vi "Vision Processing.vi"(4 "yaw":dbl, 6 "Line Border":cluster{"Top":dbl, "Bottom":dbl}={"Top"=6.0, "Bottom"=1.0}, 7 "LED Color":T5={"Hue"={107.81818389892578, 139.81818389892578}, "Sat"={176.07142857142858, 255.0}, "Val"={40.53571428571429, 255.0}} {"Hue" scale=0.0..255.0 scale format="%#_3g"}, 8 "Score Cutoff %":dbl=70.0, 9 "Masked Image":T1, 10 "Boiler?":bool, 11 "New Image":T1) -> (1 "Original Image":T1(plugin-control), 2 "Results":T4 {"Score" format="%#_3g"; "Pixels"."Rectangle"."Numeric 5" format="%#_3g"; "Pixels"."Rectangle"."Numeric 3" format="%#_3g"; "Pixels"."Rectangle"."Numeric 2" format="%#_3g"; "Pixels"."Rectangle"."Numeric" format="%#_3g"; "Normalized"."Rectangle"."Numeric 5" format="%#_2g"; "Normalized"."Rectangle"."Numeric 3" format="%#_2g"; "Normalized"."Rectangle"."Numeric 2" format="%#_2g"; "Normalized"."Rectangle"."Numeric" format="%#_2g"; "Normalized"."Center"."?" format="%#_3g"; "Normalized"."Center"."?" format="%#_3g"; "Distance (ft)" format="%#_3g"}, 3 "Mask":T1(plugin-control))   [LabVIEW 2016]
uses:
  Vision Support Code/Camera Types.ctl
  <vilib>/Rock Robotics/WPI/Camera/WPI_CameraImageSize.ctl
  <vilib>/vision/Image Controls.llb/IMAQ Image.ctl
  <vilib>/Rock Robotics/Network Tables/NT Write Number.vi
  <vilib>/Rock Robotics/Network Tables/NT Write Boolean.vi
  <vilib>/vision/NI_Vision_Development_Module.lvlib
panel:
  out "Edge?":bool
  out "Time":u32
  in  "Image Size":T2=enum."320x240"
  in  "Color Mode":u16(ring)=3 items=["RGB", "HSL", "HSV", "HSI"]
  in  "Particles":dbl=5.0
  in  "Camera Type":T3=enum."MS HD3000 640x480"
  out "Qualified Particles":i32
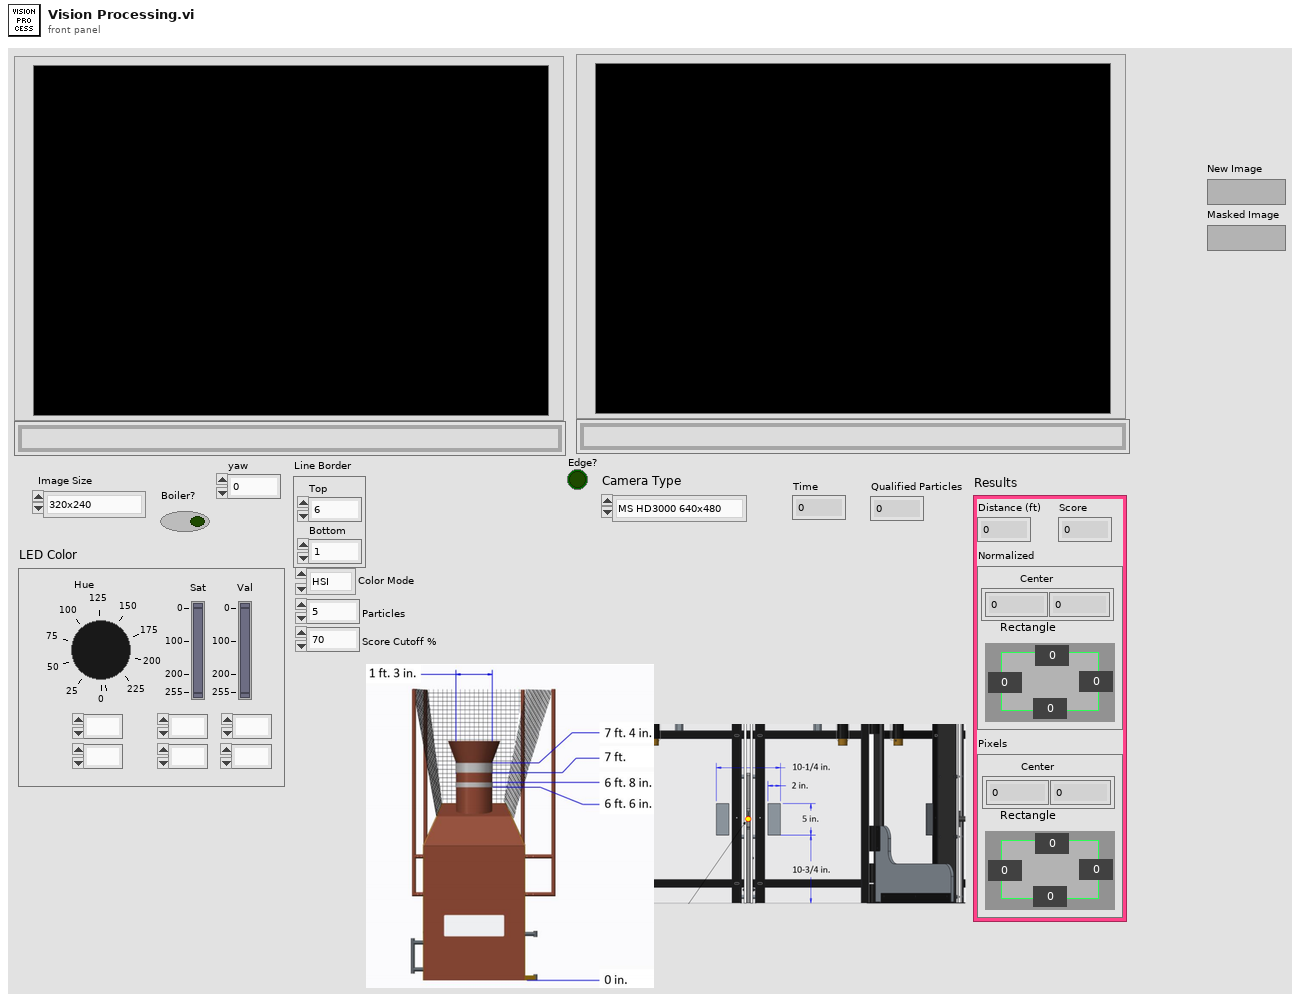
[diagram p1: front panel]
types:
  T1 = typedef "IMAQ Image.ctl" = refnum<image>
  T2 = typedef "WPI_CameraImageSize.ctl" = enum16{"640x480", "320x240", "160x120", "Custom"}
  T3 = typedef "Camera Types.ctl" = enum16{"206", "1011", "1013", "MS HD3000 square", "MS HD3000 640x480"}
  T4 = cluster{"Distance (ft)":dbl, "Score":dbl, "Normalized":cluster{"Center":cluster{dbl, dbl}, "Rectangle":cluster{"Numeric":dbl, "Numeric 2":dbl, "Numeric 3":dbl, "Numeric 5":dbl}}, "Pixels":cluster{"Center":cluster{dbl, dbl}, "Rectangle":cluster{"Numeric":dbl, "Numeric 2":dbl, "Numeric 3":dbl, "Numeric 5":dbl}}}
  T5 = cluster{"Hue":cluster{dbl, dbl}, "Sat":cluster{dbl, dbl}, "Val":cluster{dbl, dbl}}
  T6 = typedef "Particle Parameters" = i32
  T7 = cluster{"Left":dbl, "Top":dbl, "Right":dbl, "Bottom":dbl}
  T8 = cluster{"Distance (ft)":dbl, "Score":dbl, "Normalized":cluster{"Center":cluster{dbl, dbl}, "Rectangle":cluster{"Numeric":dbl, "Numeric 2":dbl, "Numeric 3":dbl, "Numeric 5":dbl}}, "Pixels":cluster{"Center":cluster{dbl, dbl}, "Rectangle":cluster{"Numeric":dbl, "Numeric 2":dbl, "Numeric 3":dbl, "Numeric 5":dbl}}}[]
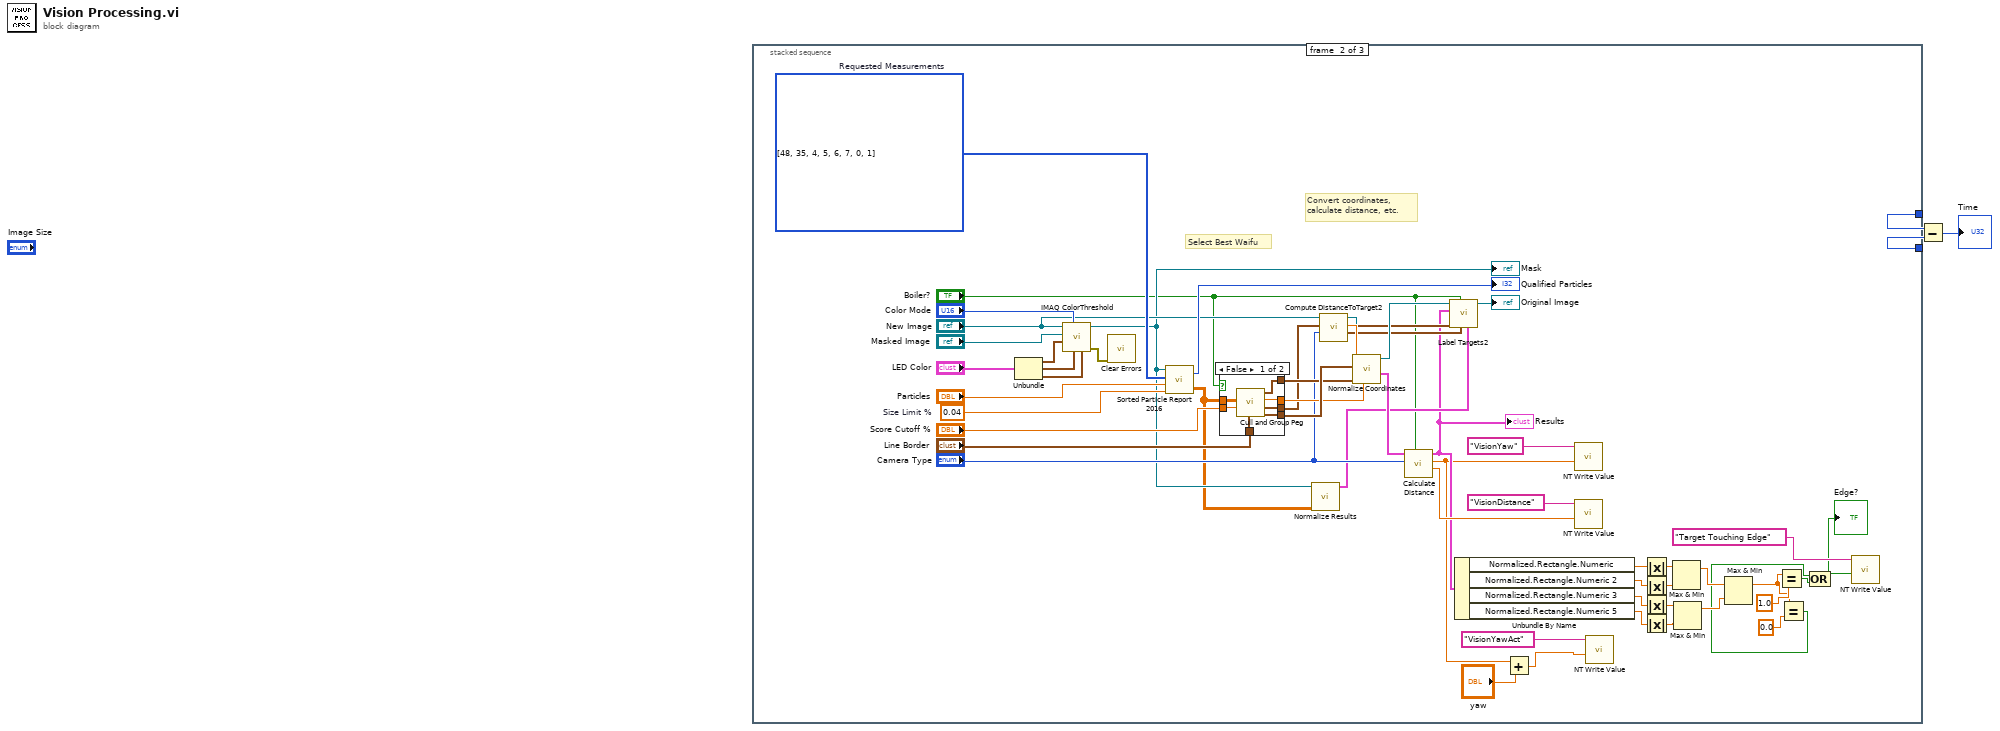
[diagram p0: block diagram]
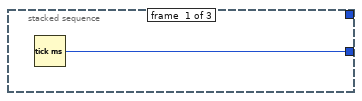
[diagram p2: hidden frame]
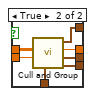
[diagram p3: hidden frame]
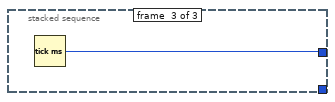
[diagram p4: hidden frame]
diagram:
  n1 = stacked-sequence {
    tunnel: [w4 _ _] -> w2
    tunnel: [_ _ w73] -> w3
    frame #0 {
      n2 = Tick Count (ms)() -> (millisecond timer value=w4:u32)
    }
    frame #1 {
      w39 = T6[] [48, 35, 4, 5, 6, 7, 0, 1] items=["Center of Mass X", "Center of Mass Y", "First Pixel X", "First Pixel Y", "Bounding Rect Left", "Bounding Rect Top", "Bounding Rect Right", "Bounding Rect Bottom", "Max Feret Diameter Start X", "Max Feret Diameter Start Y", "Max Feret Diameter End X", "Max Feret Diameter End Y", "Max Horiz. Segment Length Left", "Max Horiz. Segment Length Right", "Max Horiz. Segment Length Row", "-", "Bounding Rect Width", "Bounding Rect Height", "Bounding Rect Diagonal", "Perimeter", "Convex Hull Perimeter", "Holes' Perimeter", "Max Feret Diameter", "Equivalent Ellipse Major Axis", "Equivalent Ellipse Minor Axis", "Equivalent Ellipse Minor Axis (Feret)", "Equivalent Rect Long Side", "Equivalent Rect Short Side", "Equivalent Rect Diagonal", "Equivalent Rect Short Side (Feret)", "Average Horiz. Segment Length", "Average Vert. Segment Length", "Hydraulic Radius", "Waddel Disk Diameter", "-", "Area", "Holes' Area", "Particle & Holes' Area", "Convex Hull Area", "Image Area", "-", "Number of Holes", "Number of Horiz. Segments", "Number of Vert. Segments", "-", "Orientation", "Max Feret Diameter Orientation", "-", "% Area/Image Area", "% Area/(Particle & Holes' Area)", "Ratio of Equivalent Ellipse Axes", "Ratio of Equivalent Rect Sides", "-", "Elongation Factor", "Compactness Factor", "Heywood Circularity Factor", "Type Factor", "-", "Sum X", "Sum Y", "Sum XX", "Sum XY", "Sum YY", "Sum XXX", "Sum XXY", "Sum XYY", "Sum YYY", "-", "Moment of Inertia XX", "Moment of Inertia XY", "Moment of Inertia YY", "Moment of Inertia XXX", "Moment of Inertia XXY", "Moment of Inertia XYY", "Moment of Inertia YYY", "Norm. Moment of Inertia XX", "Norm. Moment of Inertia XY", "Norm. Moment of Inertia YY", "Norm. Moment of Inertia XXX", "Norm. Moment of Inertia XXY", "Norm. Moment of Inertia XYY", "Norm. Moment of Inertia YYY", "Hu Moment 1", "Hu Moment 2", "Hu Moment 3", "Hu Moment 4", "Hu Moment 5", "Hu Moment 6", "Hu Moment 7"]  # Requested Measurements
      w54 = 0.04  # Size Limit %
      # "Convert coordinates,\ncalculate distance, etc."
      # "Select Best Waifu"
      n3 = Unbundle("LED Color") -> ("Hue"=w58:cluster{dbl, dbl}, "Sat"=w57:cluster{dbl, dbl}, "Val"=w56:cluster{dbl, dbl})
      n4 = call "IMAQ ColorThreshold"("Blue or Luma or Val or Inten Range"=w56, "Green or Sat Range"=w57, "Color Mode"="Color Mode", "Red or Hue Range"=w58, "Image Dst"="Masked Image", "Image Src"="New Image") -> ("error out"=w53:errorcluster, "Image Dst Out"=w30:T1)  [unwired: 4 in]
      "Mask" <- w30
      n5 = call <vilib>:"Clear Errors.vi"("error in (no error)"=w53) -> ()  [unwired: 5 in, 2 out]
      n6 = call "Sorted Particle Report 2016.vi"("Min Area Size %"=w54, "Particle Count Limit"="Particles", "Pixel Measurements"=w39, "Image in"=w30) -> ("Sorted Data"=w29:dbl[][], "Particles"=→"Qualified Particles":i32)
      n7 = case shown="False" "Boiler?" {
        tunnel: "Score Cutoff %" -> [w64 w72]
        tunnel: [w59 w71] -> w50
        tunnel: [w62 w70] -> w46
        tunnel: [w61 w69] -> w45
        tunnel: [w60 w68] -> w42
        tunnel: "Line Border" -> [w65 w67]
        tunnel: w29 -> [w63 w66]
        frame False {
          n8 = call "Cull and Group Peg.vi"("Line Border"=w65, "Score Cutoff"=w64, "Sorted Data"=w63) -> ("Rect"=w59:T7, "Line"=w60:T7, "Score"=w61:dbl, "Center"=w62:cluster{"X":dbl, "Y":dbl})  [unwired: 5 in]
        }
        frame True {
          n9 = call "Cull and Group.vi"("Line Border"=w67, "Score Cutoff"=w72, "Sorted Data"=w66) -> ("Rect"=w71:T7, "Line"=w68:T7, "Score"=w69:dbl, "Center"=w70:cluster{"X":dbl, "Y":dbl})  [unwired: 5 in]
        }
      }
      n10 = call "Normalize Results.vi"("Sorted Data"=w29, "Image in"=w30) -> ("Results"=w28:T8)  [unwired: 9 in]
      n11 = call "Compute DistanceToTarget2.vi"("Camera Type"="Camera Type", "Line"=w42, "Image Src"="New Image") -> ("Edges"=w41:cluster{"X":sgl, "Y":sgl}[], "Distance (ft)"=w49:dbl, "Image Dst Out"=w48:T1)  [unwired: 6 in]
      n12 = call "Normalize Coordinates.vi"("Score"=w45, "Center"=w46, "Distance"=w49, "Bounding box"=w50, "Image in"=w48) -> ("Results"=w35:T4, "Image out"=w47:T1)  [unwired: 5 in]
      n13 = call "Calculate Distance.vi"("Boiler Mode"="Boiler?", "Camera Type"="Camera Type", "Results (in)"=w35) -> ("Average Distance"=w32:dbl, "Yaw Angle"=w12:dbl, "Results (out)"=w26:T4)  [unwired: 6 in]
      "Results" <- w26
      n14 = call "Label Targets2.vi"("Particle Results"=w28, "Edges"=w41, "Boiler?"="Boiler?", "Line"=w42, "Results"=w26, "Image in"=w47) -> ("Image out"=→"Original Image":T1)  [unwired: 5 in]
      n15 = Unbundle By Name(w26) -> ("Normalized.Rectangle.Numeric"=w24:dbl, "Normalized.Rectangle.Numeric 2"=w25:dbl, "Normalized.Rectangle.Numeric 3"=w23:dbl, "Normalized.Rectangle.Numeric 5"=w22:dbl)
      n16 = Add(x=w12, y="yaw") -> (x+y=w11:dbl)
      n17 = call-poly <vilib>:"NT Write Value.vi"("Numeric"=w12, "Name"="VisionYaw") -> ()  [unwired: 9 in, 1 out]
      n18 = call-poly <vilib>:"NT Write Value.vi"("Numeric"=w32, "Name"="VisionDistance") -> ()  [unwired: 9 in, 1 out]
      n19 = call-poly <vilib>:"NT Write Value.vi"("Numeric"=w11, "Name"="VisionYawAct") -> ()  [unwired: 9 in, 1 out]
      n20 = Absolute Value(x=w24) -> (abs(x)=w21:dbl)
      n21 = Absolute Value(x=w25) -> (abs(x)=w20:dbl)
      n22 = Absolute Value(x=w23) -> (abs(x)=w19:dbl)
      n23 = Absolute Value(x=w22) -> (abs(x)=w18:dbl)
      n24 = Max & Min(x=w21, y=w20) -> (max(x,y)=w17:dbl)  [unwired: 1 out]
      n25 = Max & Min(x=w19, y=w18) -> (max(x,y)=w16:dbl)  [unwired: 1 out]
      n26 = Max & Min(x=w17, y=w16) -> (max(x,y)=w8:dbl)  [unwired: 1 out]
      n27 = Equal?(x=w8, y=1.0) -> (x = y?=w14:bool)
      n28 = Equal?(x=w8, y=0.0) -> (x = y?=w5:bool)
      n29 = Compound Arithmetic op=OR(w5, w14) -> (w6:bool)
      "Edge?" <- w6
      n30 = call-poly <vilib>:"NT Write Value.vi"("Boolean"=w6, "Name"="Target Touching Edge") -> ()  [unwired: 9 in, 1 out]
    }
    frame #2 {
      n31 = Tick Count (ms)() -> (millisecond timer value=w73:u32)
    }
  }
  n32 = Subtract(x=w3, y=w2) -> (x-y=→"Time":u32)
